vi "Eye (SubVI).vi"(0 "Error In in":errorcluster, 1 "Error In 7":errorcluster, 5 "error in (no error)":errorcluster) -> (8 "Number_of_elements in status":dbl, 9 "Array 2":i32[](array[numeric]), 10 "Number_of_elements in notes":dbl, 11 "Notes":i32[](array[numeric]), 12 "Status":i32[](array[numeric]), 13 "Time":dbl[](array[numeric]), 14 "Array 3":dbl[](array[numeric]), 15 "Error Out 2":errorcluster, 16 "Array":i32[](array[numeric]), 17 "Error Out 7":errorcluster, 18 "Number_of_elements in time":dbl, 19 "error out":errorcluster)   [LabVIEW 2017]
uses:
  SONG.vi
panel:
  out "concatenated string":string
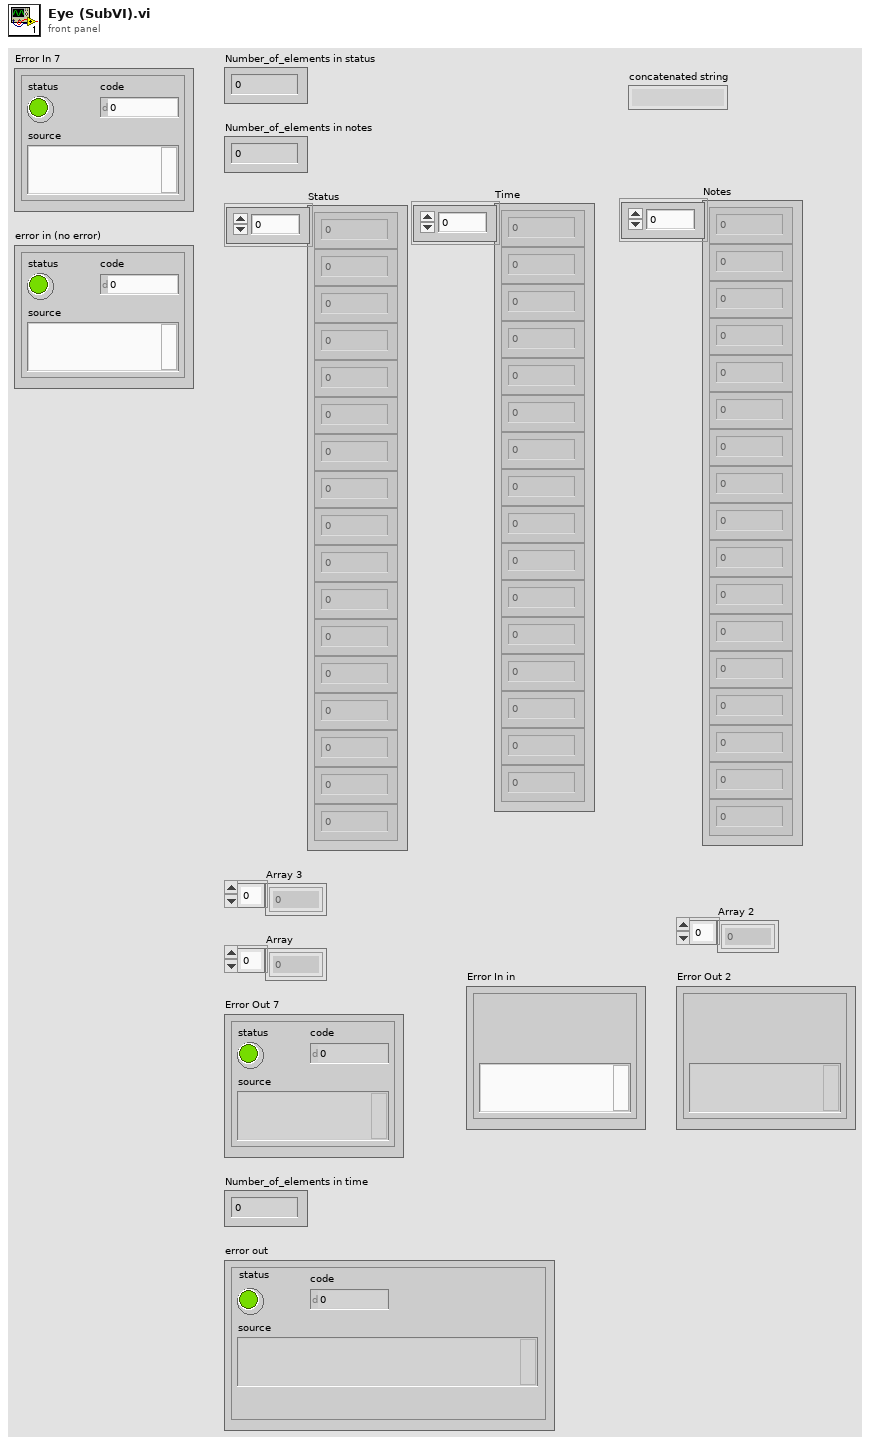
[diagram p1: front panel]
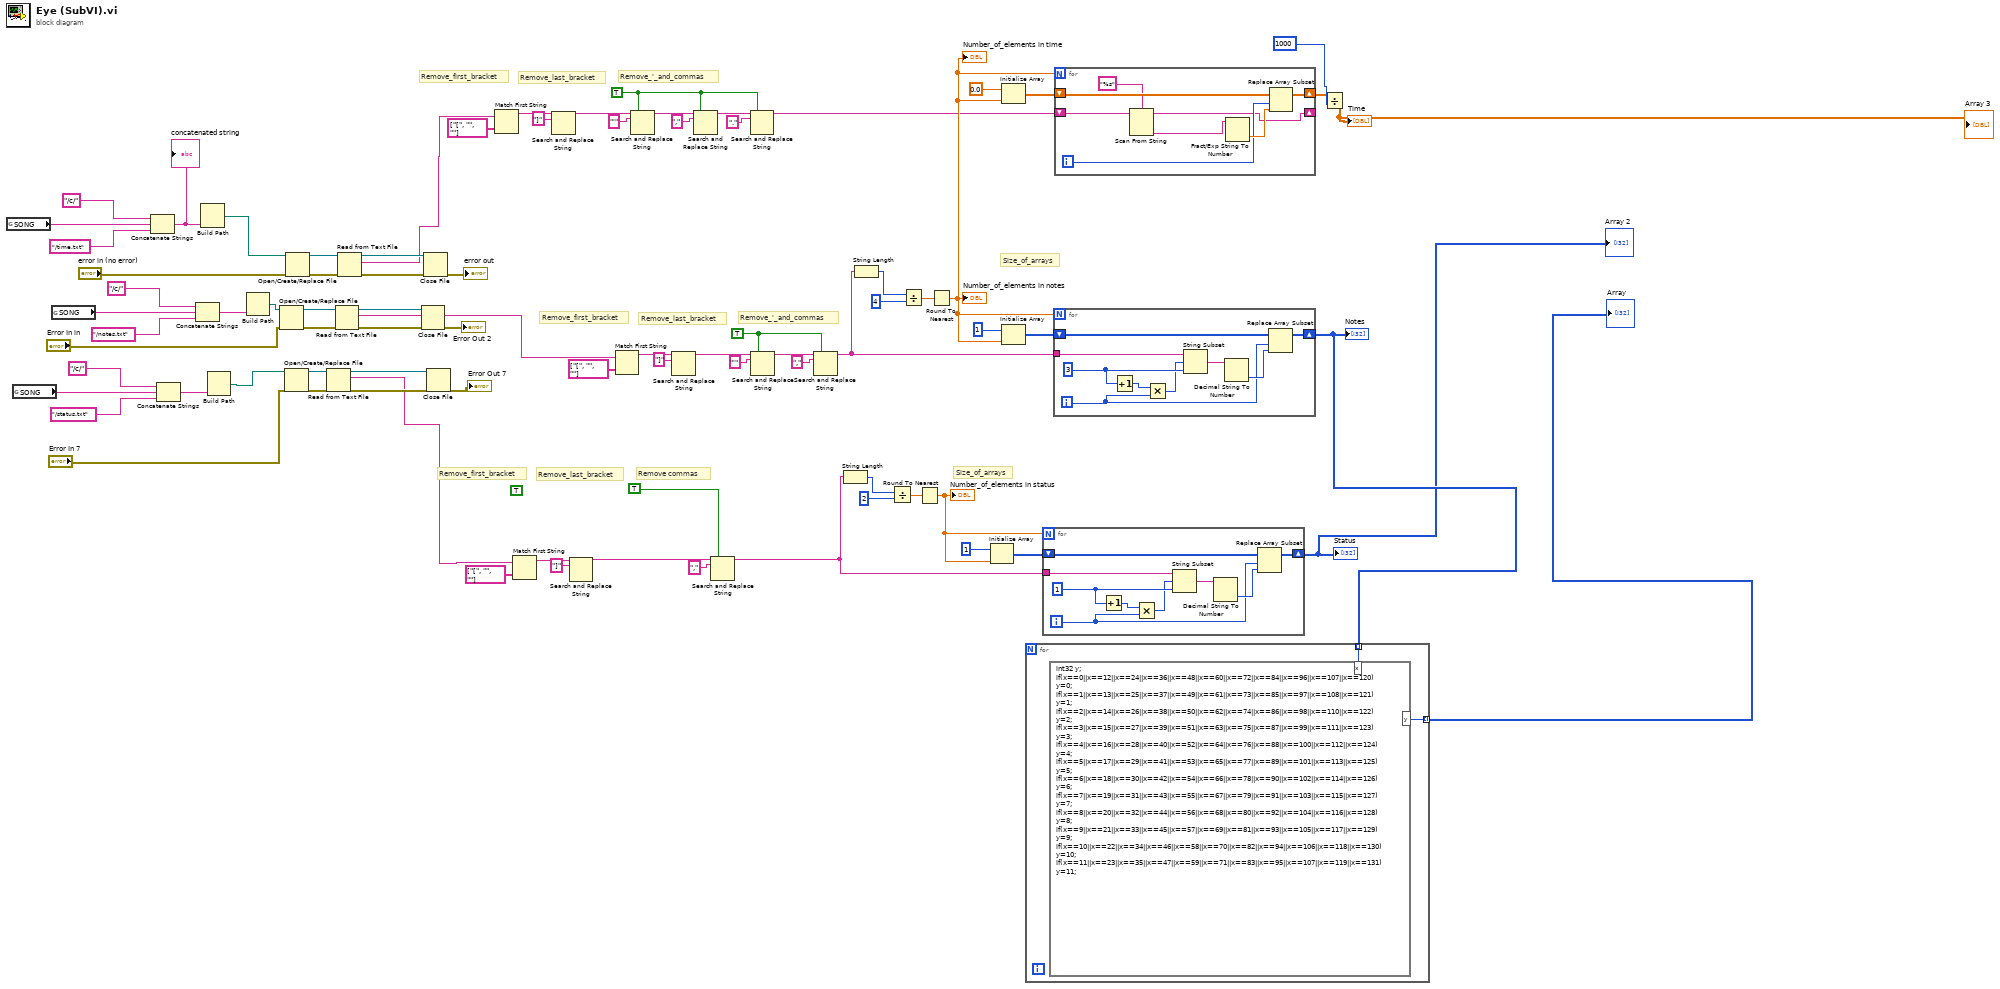
[diagram p0: block diagram]
diagram:
  (unwired) TRUE ("replace all? (F)")
  w28 = TRUE ("replace all? (F)")
  w42 = TRUE ("replace all? (F)")
  # "Size_of_arrays"
  # "Remove commas"
  # "Remove_last_bracket"
  # "Remove_first_bracket"
  # "Remove_'_and_commas"
  # "Remove_last_bracket"
  # "Remove_first_bracket"
  # "Size_of_arrays"
  # "Remove_'_and_commas"
  # "Remove_last_bracket"
  # "Remove_first_bracket"
  n1 = global read "SONG.vi" "SONG"() -> (w14:string)
  n2 = global read "SONG.vi" "SONG"() -> (w4:string)
  n3 = global read "SONG.vi" "SONG"() -> (w9:string)
  n4 = Concatenate Strings("/c/" ("string"), w14, "/time.txt" ("string")) -> (w12:string)
  "concatenated string" <- w12
  n5 = Concatenate Strings("/c/" ("string"), w4, "/status.txt" ("string")) -> (w2:string)
  n6 = Concatenate Strings("/c/" ("string"), w9, "/notes.txt" ("string")) -> (w7:string)
  n7 = Build Path(name or relative path=w12) -> (appended path=w11:path)  [unwired: 1 in]
  n8 = Build Path(name or relative path=w2) -> (appended path=w1:path)  [unwired: 1 in]
  n9 = Build Path(name or relative path=w7) -> (appended path=w6:path)  [unwired: 1 in]
  n10 = Open/Create/Replace File(file path (use dialog)=w6, error in="Error In in") -> (refnum out=w77:refnum<file>, error out=w78:errorcluster)  [unwired: 4 in, 1 out]
  n11 = Open/Create/Replace File(file path (use dialog)=w1, error in="Error In 7") -> (refnum out=w80:refnum<file>, error out=w79:errorcluster)  [unwired: 4 in, 1 out]
  n12 = Open/Create/Replace File(file path (use dialog)=w11, error in="error in (no error)") -> (refnum out=w70:refnum<file>, error out=w69:errorcluster)  [unwired: 4 in, 1 out]
  n13 = Read from Text File(file (use dialog)=w80, error in=w79) -> (refnum out=w82:refnum<file>, text=w64:string, error out=w81:errorcluster)  [unwired: 2 in, 1 out]
  n14 = Read from Text File(file (use dialog)=w77, error in=w78) -> (refnum out=w74:refnum<file>, text=w48:string, error out=w75:errorcluster)  [unwired: 2 in, 1 out]
  n15 = Read from Text File(file (use dialog)=w70, error in=w69) -> (refnum out=w73:refnum<file>, text=w46:string, error out=w72:errorcluster)  [unwired: 2 in, 1 out]
  n16 = Close File(refnum=w74, error in=w75) -> (error out=→"Error Out 2":errorcluster)  [unwired: 1 out]
  n17 = Close File(refnum=w73, error in=w72) -> (error out=→"error out":errorcluster)  [unwired: 1 out]
  n18 = Close File(refnum=w82, error in=w81) -> (error out=→"Error Out 7":errorcluster)  [unwired: 1 out]
  n19 = Match First String(2:string[] ["[", "", ""] ("string array"), 3:w46) -> (1:w17:string)  [unwired: 1 out]
  n20 = Match First String(2:string[] ["[", "", ""] ("string array"), 3:w64) -> (1:w53:string)  [unwired: 1 out]
  n21 = Search and Replace String(input string=w17, search string="]") -> (result string=w19:string)  [unwired: 6 in, 3 out]
  n22 = Search and Replace String(input string=w53, search string="]") -> (result string=w55:string)  [unwired: 6 in, 3 out]
  n23 = Match First String(2:string[] ["[", "", ""] ("string array"), 3:w48) -> (1:w37:string)  [unwired: 1 out]
  n24 = Search and Replace String(replace all?=w42, input string=w19, search string="'") -> (result string=w22:string)  [unwired: 5 in, 3 out]
  n25 = Search and Replace String(input string=w37, search string="]") -> (result string=w35:string)  [unwired: 6 in, 3 out]
  n26 = Search and Replace String(replace all?=w42, input string=w22, search string=",") -> (result string=w39:string)  [unwired: 5 in, 3 out]
  n27 = Search and Replace String(replace all?=TRUE ("replace all? (F)"), input string=w55, search string=",") -> (result string=w62:string)  [unwired: 5 in, 3 out]
  n28 = Search and Replace String(replace all?=w42, input string=w39, search string=".") -> (result string=w40:string)  [unwired: 5 in, 3 out]
  n29 = Search and Replace String(replace all?=w28, input string=w35, search string="'") -> (result string=w32:string)  [unwired: 5 in, 3 out]
  n30 = Search and Replace String(replace all?=w28, input string=w32, search string=",") -> (result string=w27:string)  [unwired: 5 in, 3 out]
  n31 = String Length(string=w62) -> (length=w60:i32)
  n32 = String Length(string=w27) -> (length=w31:i32)
  n33 = Divide(x=w60, y=2) -> (x/y=w58:dbl)
  n34 = Divide(x=w31, y=4) -> (x/y=w29:dbl)
  n35 = Round To Nearest(number=w58) -> (nearest integer value=w61:dbl)
  "Number_of_elements in status" <- w61
  n36 = Round To Nearest(number=w29) -> (nearest integer value=w49:dbl)
  "Number_of_elements in time" <- w49
  "Number_of_elements in notes" <- w49
  n37 = Initialize Array(1 ("Number_of_elements"), w61) -> (w56:i32[])
  n38 = Initialize Array(0.0 ("Number_of_elements"), w49) -> (w24:dbl[])
  n39 = Initialize Array(1 ("Number_of_elements"), w49) -> (w25:i32[])
  n40 = for {
    N: w61 -> [_]
    tunnel: w62 -> [w92]
    shift-right: [w84] -> w66
    shift-left: w56 -> [w87]
    i -> [w85]
    w91 = 1 ("length (rest)")
    n41 = Increment(x=w91) -> (x+1=w90:i32)
    n42 = Multiply(x=w90, y=w85) -> (x*y=w89:i32)
    n43 = String Subset(string=w92, offset (0)=w89, length (rest)=w91) -> (substring=w88:string)
    n44 = Decimal String To Number(string=w88) -> (number=w86:i32)  [unwired: 2 in, 1 out]
    n45 = Replace Array Subset(array=w87, new element=w86, index=w85) -> (w84:i32[])
  }
  "Status" <- w66
  "Array 2" <- w66
  n46 = for {
    N: w49 -> [_]
    tunnel: w27 -> [w101]
    shift-right: [w93] -> w67
    shift-left: w25 -> [w96]
    i -> [w94]
    w100 = 3 ("length (rest)")
    n47 = Increment(x=w100) -> (x+1=w99:i32)
    n48 = Multiply(x=w99, y=w94) -> (x*y=w98:i32)
    n49 = String Subset(string=w101, offset (0)=w98, length (rest)=w100) -> (substring=w97:string)
    n50 = Decimal String To Number(string=w97) -> (number=w95:i32)  [unwired: 2 in, 1 out]
    n51 = Replace Array Subset(array=w96, new element=w95, index=w94) -> (w93:i32[])
  }
  "Notes" <- w67
  n52 = for {
    tunnel: w67 -> [w103] mode=indexing
    tunnel: [w102] -> w68 mode=indexing
    n53 = formula code="int32 y;\nif(x==0||x==12||x==24||x==36||x==48||x==60||x==72||x==84||x==96||x==107||x==120)\ny=0;\nif(x==1||x==13||x==25||x==37||x==49||x==61||x==73||x==85||x==97||x==108||x==121)\ny=1;\nif(x==2||x==14||x==26||x==38||x==50||x==62||x==74||x==86||x==98||x==110||x==122)\ny=2;\nif(x==3||x==15||x==27||x==39||x==51||x==63||x==75||x==87||x==99||x==111||x==123)\ny=3;\nif(x==4||x==16||x==28||x==40||x==52||x==64||x==76||x==88||x==100||x==112||x==124)\ny=4;\nif(x==5||x==17||x==29||x==41||x==53||x==65||x==77||x==89||x==101||x==113||x==125)\ny=5;\nif(x==6||x==18||x==30||x==42||x==54||x==66||x==78||x==90||x==102||x==114||x==126)\ny=6;\nif(x==7||x==19||x==31||x==43||x==55||x==67||x==79||x==91||x==103||x==115||x==127)\ny=7;\nif(x==8||x==20||x==32||x==44||x==56||x==68||x==80||x==92||x==104||x==116||x==128)\ny=8;\nif(x==9||x==21||x==33||x==45||x==57||x==69||x==81||x==93||x==105||x==117||x==129)\ny=9;\nif(x==10||x==22||x==34||x==46||x==58||x==70||x==82||x==94||x==106||x==118||x==130)\ny=10;\nif(x==11||x==23||x==35||x==47||x==59||x==71||x==83||x==95||x==107||x==119||x==131)\ny=11;"("x"=w103) -> ("y"=w102:i32)
  }
  "Array" <- w68
  n54 = for {
    N: w49 -> [_]
    shift-right: [w108] -> w43
    shift-left: w24 -> [w111]
    shift-right: [w104] -> _
    shift-left: w40 -> [w106]
    i -> [w109]
    n55 = Scan From String(format string="%s", input string=w106) -> (remaining string=w104:string, output 1=w105:string)  [unwired: 3 in, 2 out]
    n56 = Fract/Exp String To Number(string=w105) -> (number=w110:dbl)  [unwired: 3 in, 1 out]
    n57 = Replace Array Subset(array=w111, new element=w110, index=w109) -> (w108:dbl[])
  }
  n58 = Divide(x=w43, y=1000 ("length (rest)")) -> (x/y=→"Time" →"Array 3":dbl[])
